vi "Save_Info.vi"(8 "error in (no error)":errorcluster, 11 "Class in":refnum<class "IB_MSI.lvclass">) -> (0 "error out":errorcluster, 3 "Class out":refnum<class "IB_MSI.lvclass">)   [LabVIEW 2020, in "IB_MSI.lvclass"]
uses:
  <vilib>/AppBuilder/IB_Classes/MSI/IB_MSI.lvclass
  <vilib>/AppBuilder/IB_Classes/MSI/IB_MSI.lvclass/IB_MSI.ctl
  <vilib>/AppBuilder/IB_RW_Project/IB_RW_Project_PropBag_Action.ctl
  <vilib>/AppBuilder/IB_Classes/Installer/Installer.lvclass
  e:/builds/penguin/labview/branches/2020/dev/dist/vi.lib/AppBuilder/IB_Classes/Installer/Installer.lvclass
  e:/builds/penguin/labview/branches/2020/dev/dist/vi.lib/AppBuilder/IB_Classes/MSI/IB_MSI.lvclass
  <resource>/Framework/Providers/Builds/Installer/CDK_sTypeDef_HWImportOption.ctl
  <vilib>/AppBuilder/IB_RW_Project/IB_RW_Project_MSI_Data.ctl
panel:
  in  "MSI":T1
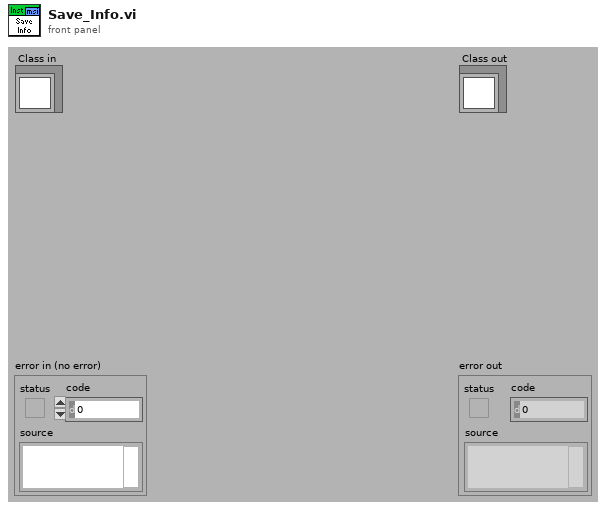
[diagram p1: front panel]
types:
  T1 = typedef "IB_RW_Project_MSI_Data.ctl" = cluster{"upgradeCode":string, "distID":string, "windowMessage":string, "windowTitle":string, "arpPhone":string, "arpContact":string, "arpURL":string, "arpCompany":string, "licenseID":string, "welcomeImageID":string, "bannerImageID":string, "osCheck":i32, "msiFileName":string, "cabFileName":string, "hwOption":T2, "hwPath":path, "winsec.certificate":string, "winsec.timestamp":string, "winsec.description":string, "autoselect drivers":bool, "hide non-runtimes":bool}
  T2 = typedef "CDK_sTypeDef_HWImportOption.ctl" = enum16{"<none>", "Merge", "Replace", "Dialog"}
  T3 = typedef "IB_RW_Project_PropBag_Action.ctl" = enum16{"read", "write", "clear", "readPrevious", "writePrevious", "clearPrevious"}
  T4 = typedef "IB_Installer.ctl" = cluster{"Destination":refnum<class "IB_Destination.lvclass">[], "Source":refnum<class "IB_Source.lvclass">[], "buildObject":T5, "defaultDir":string, "platform":string, "author":string, "productName":string, "buildSpecName":string, "hide":bool, "requireLVDevSys":bool, "autoIncrement":bool, "includeError":bool, "readmeID":string, "buildLocation":path, "readmePath":path, "mediaSize":u16, "language":T6, "productVersion":T7, "preview":bool, "programmatic":bool, "progressBarEvents":T8, "userLog_Path":path, "shortcutAddresses":T10[], "EXE_Install Address":string, "EXE_Uninstall Address":string, "additional NIPaths":refnum<class "Dest_NI_NIPath.lvclass">[], "web service itemIDs":string[], "installerName":string}
  T5 = typedef "ItemRef.ctl" = u64
  T6 = typedef "CDK_sTypeDef_Languages.ctl" = u16
  T7 = typedef "CDK_sTypeDef_ProductVersion.ctl" = cluster{"Major":u8, "Minor":u8, "Update":u16}
  T8 = typedef "provcom_ProgressBar_Events.ctl" = cluster{"newJob":refnum<user-event>, "newItem":refnum<user-event>, "errorMsg":T9, "cancel":refnum<user-event>}
  T9 = typedef "mxLvBuildError.ctl" = refnum<user-event>
  T10 = typedef "CDK_sTypeDef_ShortcutAddress.ctl" = cluster{"file":string, "shortcut":string}
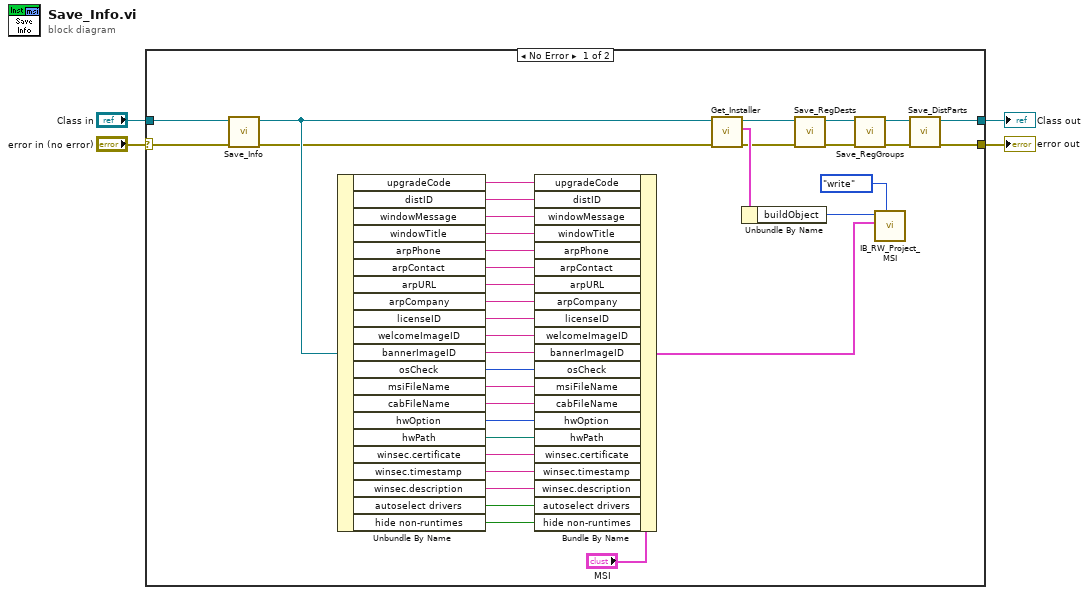
[diagram p0: block diagram]
diagram:
  n1 = case shown="No Error" "error in (no error)" {
    selector: "error in (no error)" -> [w16 w44]
    tunnel: [w21 w44] -> w4
    tunnel: [w22 w43] -> w3
    tunnel: "Class in" -> [w17 w43]
    frame No Error {
      n2 = call-parent "Save_Info.vi"("error in (no error)"=w16, "Class in"=w17) -> ("error out"=w7:errorcluster, "Class out"=w8:refnum<class "IB_MSI.lvclass">)  [unwired: 8 out]
      n3 = Unbundle By Name(w8) -> ("upgradeCode"=w41:string, "distID"=w40:string, "windowMessage"=w39:string, "windowTitle"=w38:string, "arpPhone"=w37:string, "arpContact"=w36:string, "arpURL"=w35:string, "arpCompany"=w34:string, "licenseID"=w33:string, "welcomeImageID"=w32:string, "bannerImageID"=w31:string, "osCheck"=w30:i32, "msiFileName"=w29:string, "cabFileName"=w28:string, "hwOption"=w27:T2, "hwPath"=w26:path, "winsec.certificate"=w9:string, "winsec.timestamp"=w10:string, "winsec.description"=w11:string, "autoselect drivers"=w6:bool, "hide non-runtimes"=w5:bool)
      n4 = Bundle By Name(cluster="MSI", "upgradeCode"=w41, "distID"=w40, "windowMessage"=w39, "windowTitle"=w38, "arpPhone"=w37, "arpContact"=w36, "arpURL"=w35, "arpCompany"=w34, "licenseID"=w33, "welcomeImageID"=w32, "bannerImageID"=w31, "osCheck"=w30, "msiFileName"=w29, "cabFileName"=w28, "hwOption"=w27, "hwPath"=w26, "winsec.certificate"=w9, "winsec.timestamp"=w10, "winsec.description"=w11, "autoselect drivers"=w6, "hide non-runtimes"=w5) -> (w25:T1)
      n5 = call <vilib>:"Get_Installer.vi"("error in (no error)"=w7, "Installer in"=w8) -> ("error out"=w19:errorcluster, "data"=w23:T4, "Installer out"=w20:refnum<class "IB_MSI.lvclass">)  [unwired: 7 out]
      n6 = Unbundle By Name(w23) -> ("buildObject"=w18:T5)
      n7 = call <vilib>:"Save_RegDests.vi"("error in (no error)"=w19, "Class in"=w20) -> ("error out"=w13:errorcluster, "Class out"=w15:refnum<class "IB_MSI.lvclass">)  [unwired: 8 out]
      n8 = call <vilib>:"Save_RegGroups.vi"("error in (no error)"=w13, "IB_MSI in"=w15) -> ("error out"=w12:errorcluster, "IB_MSI out"=w14:refnum<class "IB_MSI.lvclass">)  [unwired: 8 out]
      n9 = call <vilib>:"IB_RW_Project_MSI.vi"("action"=IB_RW_Project_PropBag_Action."write", "MSI in"=w25, "Object In"=w18) -> ()  [unwired: 2 in, 7 out]
      n10 = call <vilib>:"Save_DistParts.vi"("error in (no error)"=w12, "Class in"=w14) -> ("error out"=w21:errorcluster, "Class out"=w22:refnum<class "IB_MSI.lvclass">)  [unwired: 8 out]
    }
    frame Error {
    }
  }
  "error out" <- w4
  "Class out" <- w3
